vi "Get Pixel by Event Structure.vi"() -> ()   [LabVIEW 2012, in "Picture Box Tools.lvlib"]
uses:
  Picture Box Tools.lvlib
panel:
  out "Color":u32(colorbox)
  in  "停止按钮":bool
  out "Load Picture":picture caption="载入图片"
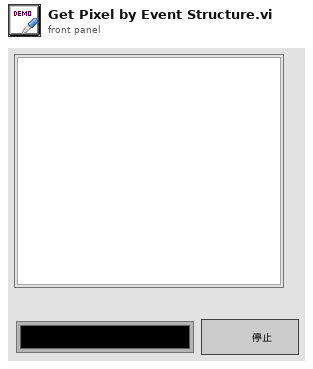
[diagram p1: front panel]
types:
  T1 = typedef "imagedata.ctl" = cluster{"image type":i32, "image depth":i32, "image":u8[], "mask":u8[], "colors":u32[], "Rectangle":cluster{"left":i16, "top":i16, "right":i16, "bottom":i16}}
  T2 = typedef "LVPoint32TypeDef.ctl" = cluster{"Horizontal":i32, "Vertical":i32}
  T3 = typedef "LVPositionTypeDef.ctl" = cluster{"Left":i32, "Top":i32}
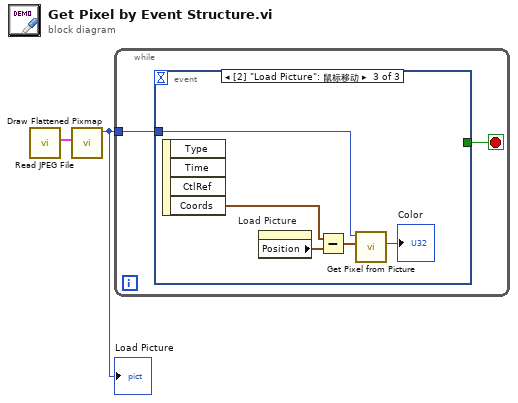
[diagram p0: block diagram]
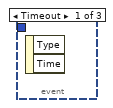
[diagram p2: hidden frame]
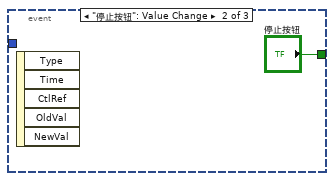
[diagram p3: hidden frame]
diagram:
  n1 = call <vilib>:"Read JPEG File.vi"() -> ("image data"=w2:T1)  [unwired: 9 in, 2 out]
  n2 = call <vilib>:"Draw Flattened Pixmap.vi"("image data"=w2) -> ("new picture"=w1:picture)  [unwired: 8 in]
  "Load Picture" <- w1
  n3 = while {
    tunnel: w1 -> [w3]
    stop <- w4 stop-if-true
    n4 = event shown="[2] \"Load Picture\": 鼠标移动" {
      selector: _ -> [_ _ _]
      dyn-events: _ -> [_ _ _]
      timeout: _ -> [_ _ _]
      tunnel: [_ "停止按钮" _] -> w4
      tunnel: w3 -> [_ _ w10]
      event Timeout {
        n5 = event-data() -> ()  [unwired: 1 in, 2 out]
      }
      event "停止按钮": Value Change {
        n6 = event-data() -> ()  [unwired: 1 in, 5 out]
      }
      event "Load Picture": Mouse Move {
        n7 = event-data() -> ("Coords"=w8:T2)  [unwired: 1 in, 3 out]
        n8 = property on="Load Picture" class="Pict"() -> ("Position"=w7:T3)  [unwired: 2 in, 2 out]
        n9 = Subtract(x=w8, y=w7) -> (x-y=w6:T2)
        n10 = call "Get Pixel from Picture.vi"("Pos"=w6, "Picture in"=w10) -> ("Color"=→"Color":u32)  [unwired: 7 in, 2 out]
      }
    }
  }
